vi "Get Channel Settings.vi"(1 "Channel Settings typedef":T1={"Name"="", "Terminal Information"={"IO Device"=enum."none", "Channel"=0, "Sensor Type"=enum."Voltage"}, "Calibration Information"={"Excitation Voltage"=1.0, "Calibration Factor"=1.0, "Zero Value"=0.0, "Calibration Formula"="(x-x0) / (Ve * CF)", "Units"="V"}}) -> (0 "Channel Settings ducktype":T4)   [LabVIEW 2021, in "Settings.lvlib"]
uses:
  Acquisition/IO Device.ctl
  Acquisition/Sensor Type.ctl
  Acquisition/Channel Settings.ctl
  Settings.lvlib
  Acquisition/Acquisition.lvlib
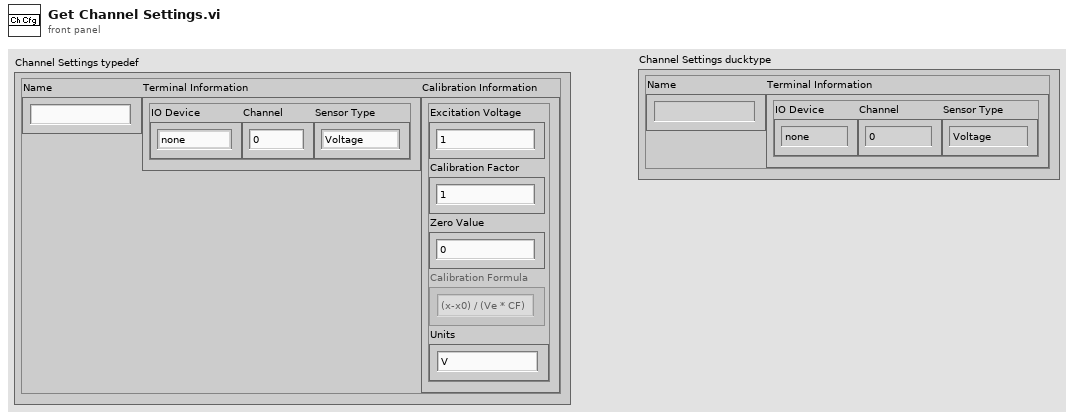
[diagram p1: front panel]
types:
  T1 = typedef "Acquisition.lvlib/Channel Settings.ctl" = cluster{"Name":string, "Terminal Information":cluster{"IO Device":T2, "Channel":i32, "Sensor Type":T3}, "Calibration Information":cluster{"Excitation Voltage":dbl, "Calibration Factor":dbl, "Zero Value":dbl, "Calibration Formula":string, "Units":string}}
  T2 = typedef "Acquisition.lvlib/IO Device.ctl" = enum16{"none", "9219", "9401"}
  T3 = typedef "Acquisition.lvlib/Sensor Type.ctl" = enum16{"Voltage", "Load", "Pressure", "Encoder"}
  T4 = cluster{"Name":string, "Terminal Information":cluster{"IO Device":T2, "Channel":i32, "Sensor Type":T3}}
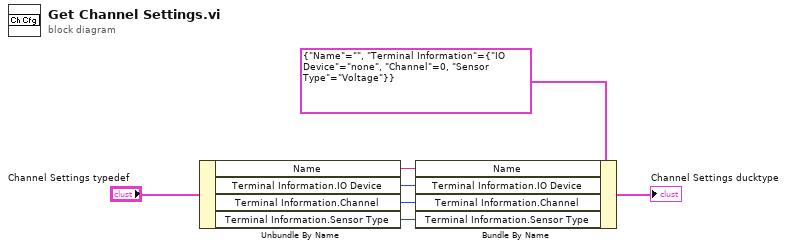
[diagram p0: block diagram]
diagram:
  n1 = Unbundle By Name("Channel Settings typedef") -> ("Name"=w7:string, "Terminal Information.IO Device"=w3:T2, "Terminal Information.Channel"=w2:i32, "Terminal Information.Sensor Type"=w1:T3)
  n2 = Bundle By Name(cluster=T4 {"Name"="", "Terminal Information"={"IO Device"=enum."none", "Channel"=0, "Sensor Type"=enum."Voltage"}} ("Channel Settings ducktype"), "Name"=w7, "Terminal Information.IO Device"=w3, "Terminal Information.Channel"=w2, "Terminal Information.Sensor Type"=w1) -> (→"Channel Settings ducktype":T4)
